vi "HWMONITOR.vi"(8 "error in":errorcluster, 10 "String":string, 11 "array":path[](array[path])) -> (0 "error out 8":errorcluster)   [LabVIEW 2025]
panel:
  out "False":string[](array[string])
  in  "Selector array":bool[](array[boolean])=[TRUE, TRUE, TRUE, TRUE, TRUE, TRUE, TRUE, TRUE, TRUE, TRUE, TRUE, FALSE, TRUE, FALSE, TRUE, FALSE, TRUE, FALSE, TRUE, FALSE, TRUE, FALSE, TRUE, FALSE, TRUE, FALSE, TRUE, FALSE, TRUE, FALSE, TRUE, TRUE]
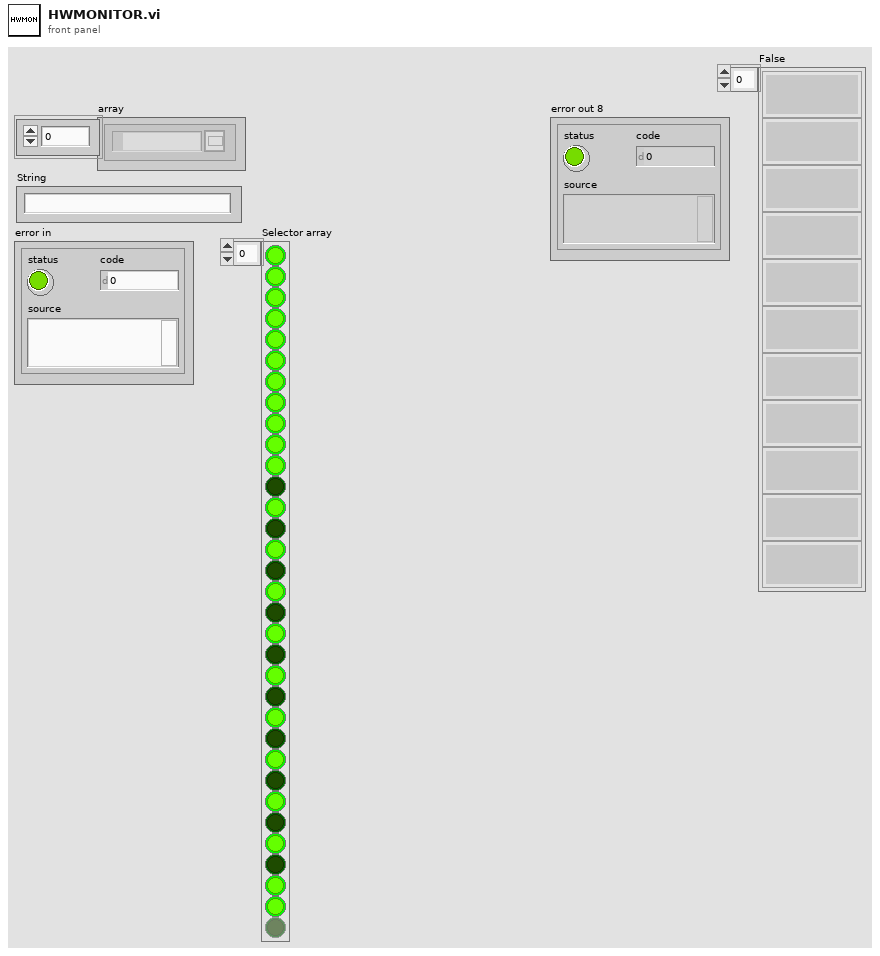
[diagram p1: front panel]
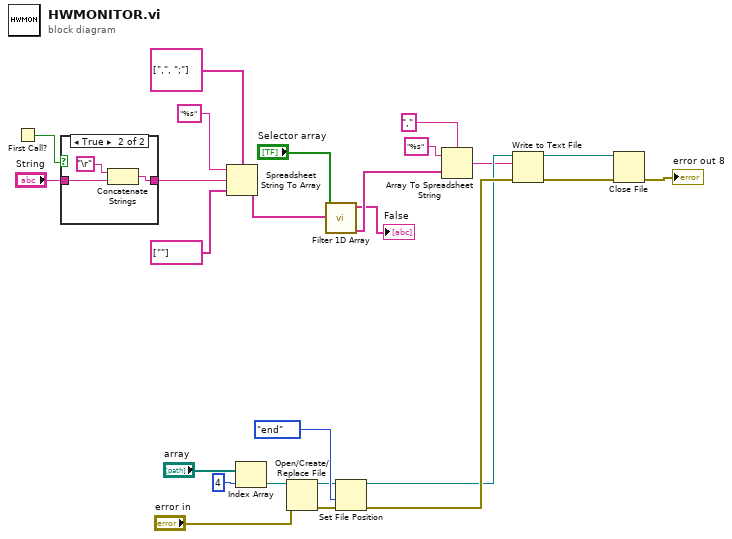
[diagram p0: block diagram]
diagram:
  n1 = First Call?() -> (First Call?: T/F=w9:bool)
  n2 = case shown="True" w9 {
    tunnel: [w26 w28] -> w8
    tunnel: "String" -> [w26 w27]
    frame False {
    }
    frame True {
      n3 = Concatenate Strings("\r", w27) -> (w28:string)
    }
  }
  n4 = Spreadsheet String To Array(delimiter (Tab)=string[] [",", ";"], format string="%s", spreadsheet string=w8, array type (2D Dbl)=string[] [""]) -> (array=w3:string[])
  n5 = Index Array(array="array", index=4 ("index (row)")) -> (element=w15:path)
  n6 = Open/Create/Replace File(file path (use dialog)=w15, error in="error in") -> (refnum out=w16:refnum<file>, error out=w19:errorcluster)  [unwired: 4 in, 1 out]
  n7 = call "Filter 1D Array.vi"("Input"=w3, "Selector array"="Selector array") -> ("True"=w2:string[], "False"=→"False":string[])  [unwired: 8 in]
  n8 = Set File Position(refnum=w16, from (0:start)=enum16{"start", "end", "current"}."end", error in=w19) -> (refnum out=w17:refnum<file>, error out=w18:errorcluster)  [unwired: 1 in]
  n9 = Array To Spreadsheet String(delimiter (Tab)=",", array=w2, 3:"%s" ("format string")) -> (spreadsheet string=w12:string)
  n10 = Write to Text File(file (use dialog)=w17, text=w12, error in=w18) -> (refnum out=w21:refnum<file>, error out=w20:errorcluster)  [unwired: 1 in, 1 out]
  n11 = Close File(refnum=w21, error in=w20) -> (error out=→"error out 8":errorcluster)  [unwired: 1 out]
